vi "[Part 1] Extract Data from N-Channel Array (1D Waveform).vi"() -> ()   [LabVIEW 2020]
uses:
  <vilib>/DAQmx/read.llb/DAQmx Read (Analog 1D Wfm NChan NSamp).vi
  <vilib>/DAQmx/create/channels.llb/DAQmx Create Channel (AI-Voltage-Basic).vi
  <vilib>/DAQmx/configure/timing.llb/DAQmx Timing (Sample Clock).vi
  <vilib>/DAQmx/miscellaneous.llb/DAQmx Fill In Error Info.vi
  <resource>/objmgr/daqmx.rc
panel:
  in  "Index":i32
  out "Actual Sample Rate (Hz)":dbl
  in  "Desired Sample Rate (Hz)":dbl=2560.0
  in  "Number of Samples":i32=256
  in  "Stop":bool
  out "All Channels":waveform(dbl)[](graph)
  out "Indexed Channel":waveform(dbl)(graph)
  in  "Physical Channels":tag="PCI-6221/ai0, PCI-6221/ai2:3"
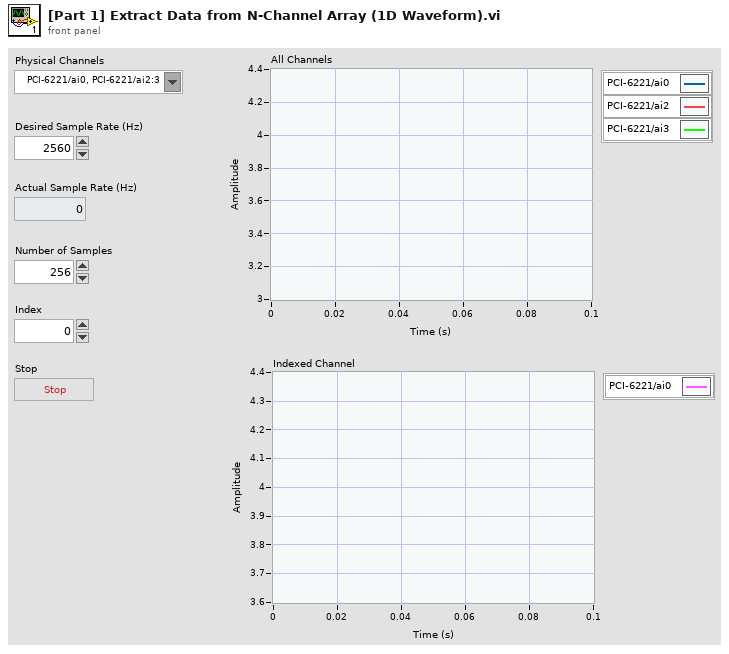
[diagram p1: front panel]
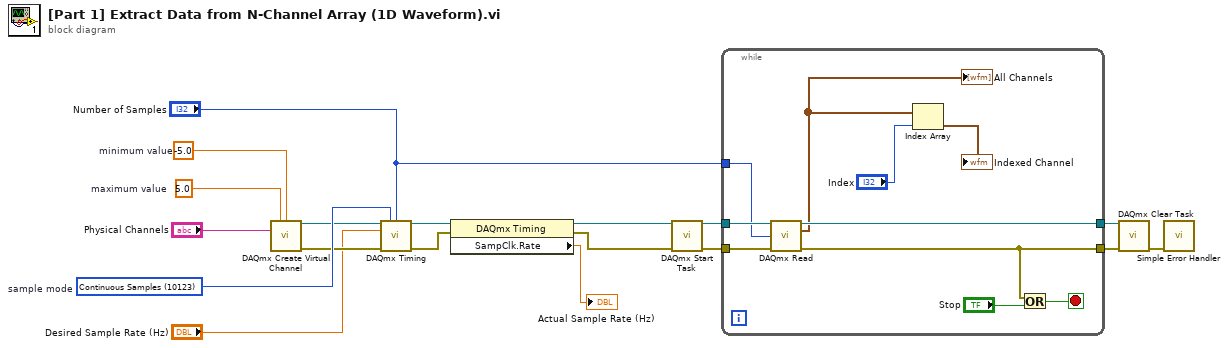
[diagram p0: block diagram]
diagram:
  w13 = 5.0  # maximum value
  w14 = -5.0  # minimum value
  w18 = 10123 items=["Finite Samples"=10178, "Continuous Samples"=10123, "Hardware Timed Single Point"=12522]  # sample mode
  n1 = call-poly <vilib>:"DAQmx Create Virtual Channel.vi"("maximum value"=w13, "minimum value"=w14, "physical channels"="Physical Channels") -> ("task out"=w17:refnum<k21>, "error out"=w16:errorcluster)  [unwired: 11 in]
  n2 = call-poly <vilib>:"DAQmx Timing.vi"("task/channels in"=w17, "sample mode"=w18, "samples per channel"="Number of Samples", "rate"="Desired Sample Rate (Hz)", "error in"=w16) -> ("task out"=w5:refnum<k21>, "error out"=w4:errorcluster)  [unwired: 9 in]
  n3 = property class="DAQmx Timing"(reference=w5, error in=w4) -> (reference out=w3:refnum<k21>, error out=w2:errorcluster, "SampClk.Rate"=→"Actual Sample Rate (Hz)":dbl)
  n4 = call <vilib>:"DAQmx Start Task.vi"("task/channels in"=w3, "error in"=w2) -> ("task out"=w9:refnum<k21>, "error out"=w8:errorcluster)  [unwired: 12 in]
  n5 = while {
    tunnel: [w28] -> w12
    tunnel: [w27] -> w11
    tunnel: w9 -> [w24]
    tunnel: w8 -> [w23]
    tunnel: "Number of Samples" -> [w22]
    stop <- w25 stop-if-true
    n6 = call-poly <vilib>:"DAQmx Read.vi"("task/channels in"=w24, "number of samples per channel"=w22, "error in"=w23) -> ("task out"=w28:refnum<k21>, "data"=w20:waveform(dbl)[], "error out"=w27:errorcluster)  [unwired: 10 in]
    "All Channels" <- w20
    n7 = Index Array "Index Array"(array=w20, index="Index") -> (element=→"Indexed Channel":waveform(dbl))
    n8 = Or(x=w27, y="Stop") -> (x .or. y?=w25:bool)
  }
  n9 = call <vilib>:"DAQmx Clear Task.vi"("task in"=w12, "error in"=w11) -> ("error out"=w10:errorcluster)  [unwired: 13 in]
  n10 = call <vilib>:"Simple Error Handler.vi"("error in (no error)"=w10) -> ()  [unwired: 4 in, 5 out]
